vi "Motion_Home Loader.vi"(8 "error in":errorcluster, 10 "timeout (60s)":dbl[unit]=60.0 caption="Time Target (s)" format="%.1f", 11 "TCP address:port":string="192.168.0.3:502") -> (0 "error out":errorcluster, 2 "elapsed time":dbl[unit]=nan format="%.1f")   [LabVIEW 2010]
uses:
  Motion_Coils Typedef.ctl
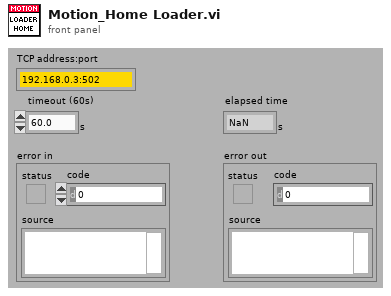
[diagram p1: front panel]
types:
  T1 = typedef "Motion_Coils Typedef.ctl" = u16
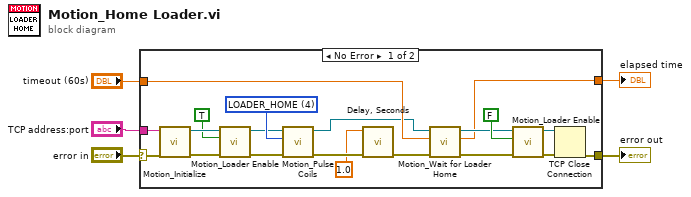
[diagram p0: block diagram]
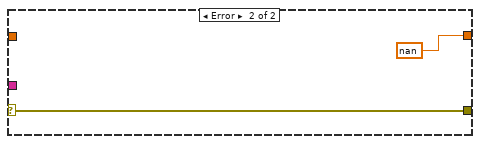
[diagram p2: hidden frame]
diagram:
  n1 = case shown="No Error" "error in" {
    selector: "error in" -> [w23 w27]
    tunnel: [w25 w27] -> w5
    tunnel: "TCP address:port" -> [w24 _]
    tunnel: [w6 dbl[unit] nan ("elapsed time")] -> w2
    tunnel: "timeout (60s)" -> [w9 _]
    frame No Error {
      w22 = T1 4 items=["GANTRY_ALARM_CLEAR", "GANTRY_ENABLE", "GANTRY_HOME", "GANTRY_GOTO", "LOADER_HOME", "LOADER_ALARM_CLEAR", "LOADER_ENABLE", "LOADER_GOTO_CONNECT", "LOADER_GOTO_LOAD", "LOADER_STOP"] ("Pulse Coil")
      n2 = call "Motion_Initialize.vi"("error in"=w23, "TCP address:port (192.168.0.3:502)"=w24) -> ("error out"=w19:errorcluster, "connection ID"=w17:refnum<k5>)  [unwired: 8 in]
      n3 = call "Motion_Loader Enable.vi"("error in (no error)"=w19, "Enable? (T)"=TRUE, "TCP Connection Refnum in"=w17) -> ("error out"=w18:errorcluster, "TCP Connection Refnum (dup)"=w16:refnum<k5>)  [unwired: 7 in]
      n4 = call "Motion_Pulse Coils.vi"("error in"=w18, "Pulse Coil"=w22, "TCP refnum"=w16) -> ("error out"=w21:errorcluster, "TCP refnum dup"=w8:refnum<k5>)  [unwired: 7 in]
      n5 = call "Delay, Seconds.vi"("error in"=w21, "delay"=dbl[unit] 1.0) -> ("error out"=w11:errorcluster)  [unwired: 5 in, 1 out]
      n6 = call "Motion_Wait for Loader Home.vi"("error in"=w11, "timeout (60s)"=w9, "TCP refnum"=w8) -> ("error out"=w10:errorcluster, "elapsed time"=w6:dbl[unit], "TCP refnum dup"=w7:refnum<k5>)  [unwired: 3 in, 3 out]
      n7 = call "Motion_Loader Enable.vi"("error in (no error)"=w10, "Enable? (T)"=FALSE, "TCP Connection Refnum in"=w7) -> ("error out"=w13:errorcluster, "TCP Connection Refnum (dup)"=w14:refnum<k5>)  [unwired: 7 in]
      n8 = TCP Close Connection(connection ID=w14, error in (no error)=w13) -> (error out=w25:errorcluster)  [unwired: 1 in, 1 out]
    }
    frame Error {
    }
  }
  "error out" <- w5
  "elapsed time" <- w2
